vi "Edgertronic_Cancel.vi"(3 "error in (no error)":errorcluster, 5 "URL":string="192.168.1.101") -> (0 "error out":errorcluster)   [LabVIEW 2015]
doc: "This VI returns a URL redirect to the actual JPEG image."
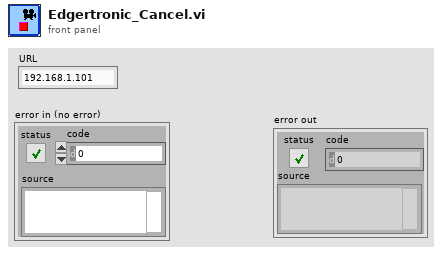
[diagram p1: front panel]
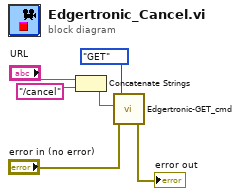
[diagram p0: block diagram]
diagram:
  n1 = Concatenate Strings("URL", "/cancel" ("GET Cmd")) -> (w3:string)
  n2 = call "Edgertronic-GET_cmd.vi"("error in (no error)"="error in (no error)", "URL"=w3, "Type"=enum16{"GET", "POST"}."GET") -> ("error out"=→"error out":errorcluster)  [unwired: 1 in, 2 out]
